vi "拉取版本信息.vi"(8 "error in (no error)":errorcluster, 11 "远端地址":string="/UP/OneStation/V4/版本升级文档.txt") -> (0 "error out":errorcluster, 3 "版本信息":cluster{"版本号":string, "更新内容":string}[](array[cluster]))   [LabVIEW 2016, in "数据传输系统.lvlib" / "update.lvlib"]
uses:
  update.lvlib
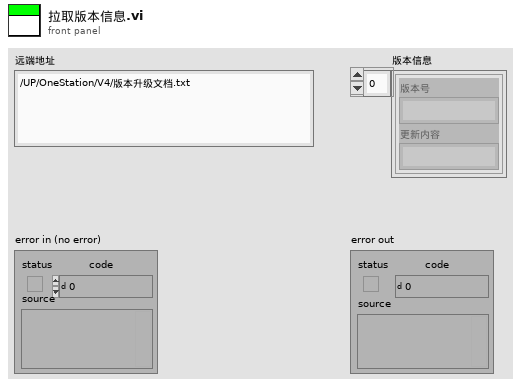
[diagram p1: front panel]
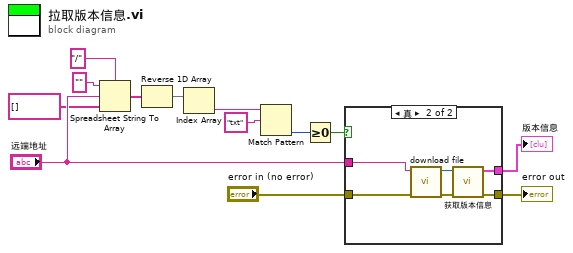
[diagram p0: block diagram]
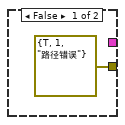
[diagram p2: hidden frame]
diagram:
  n1 = Spreadsheet String To Array(delimiter (Tab)="/" ("分隔符(Tab)"), format string="" ("格式字符串"), spreadsheet string="远端地址", array type (2D Dbl)=string[] []) -> (array=w6:string[])
  n2 = Reverse 1D Array(array=w6) -> (reversed array=w5:string[])
  n3 = Index Array(array=w5) -> (element=w4:string)  [unwired: 1 in]
  n4 = Match Pattern(string=w4, regular expression="txt" ("正则表达式")) -> (offset past match=w2:i32)  [unwired: 1 in, 3 out]
  n5 = Greater Or Equal To 0?(x=w2) -> (x >= 0?=w1:bool)
  n6 = case shown="真" w1 {
    tunnel: "error in (no error)" -> [_ w18]
    tunnel: [errorcluster {"status"=TRUE, "code"=1, "source"="路径错误"} ("error out") w17] -> w12
    tunnel: [_ w16] -> w11
    tunnel: "远端地址" -> [_ w15]
    frame False {
    }
    frame True {
      n7 = call "download file.vi"("error in (no error)"=w18, "远端地址"=w15) -> ("error out"=w19:errorcluster, "local file path"=w20:path)  [unwired: 8 in]
      n8 = call "获取版本信息.vi"("error in (no error)"=w19, "file path"=w20) -> ("error out"=w17:errorcluster, "版本信息"=w16:cluster{"版本号":string, "更新内容":string}[])  [unwired: 8 in]
    }
  }
  "error out" <- w12
  "版本信息" <- w11
